vi "main.vi"() -> ()   [LabVIEW 2023]
uses:
  <vilib>/Analysis/1siggen.llb/Ramp Pattern by Samples.vi
  <vilib>/Analysis/NI_AALBase.lvlib
panel:
  in  "save":bool
  in  "Select temp":dbl=300.0 min=2.0 max=1800.0 format="%.2g"
  out "Signal (in uV/K)":dbl format="%.3g"
  out "S, -wire  /uV":dbl format="%.3g"
  out "S, +wire /uV":dbl format="%.3g"
  out "XY Graph":cluster{"temp /K":dbl[], "S_couple":dbl[]}[](graph)
  in  "Th  (Seebeck)":u16(ring)=5 caption="Thermocouple type" items=["B", "E", "J", "K", "R", "S", "T", "N"]
  in  "points":u16=100 min=1 max=2048
  in  "end temp /K":dbl=1273.0 min=2.0 max=1800.0 format="%#.2f"
  in  "start temp /K":dbl=273.0 min=2.0 max=1800.0 format="%#.2f"
  in  "exit":bool
  # "A simple program to calculate some Seebeck coefficients. Values taken from NIST monograph 175.\nN. Dragoe, Univ Paris-Saclay (first version LV8.6, may 2005. This version was compiled on 28/06/2025)."
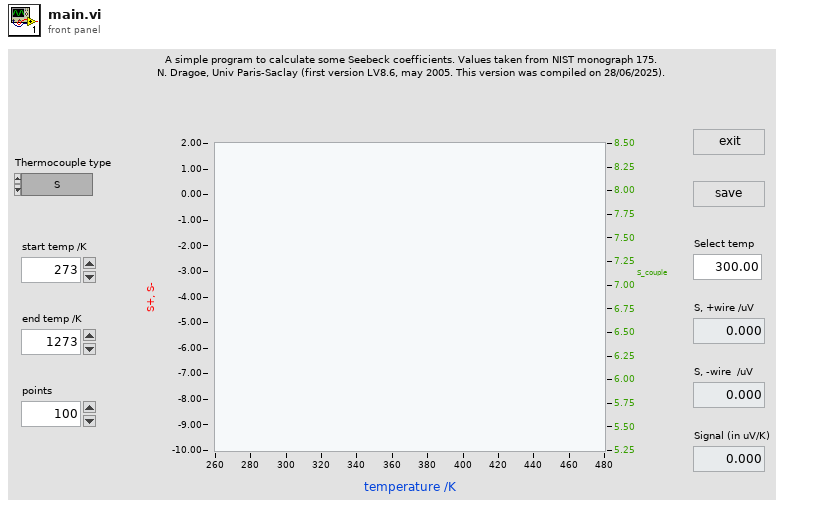
[diagram p1: front panel]
types:
  T1 = enum32{"Invalid", "Standard", "Closed", "Hidden", "Minimized", "Maximized"}
  T2 = enum32{"invalid app kind", "Development System", "Run Time System", "Student Edition", "Embedded LabVIEW", "Evaluation", "Custom"}
  T3 = cluster{"Core":cluster{"Current VI Reference":refnum<vi>, "Close Panel on Exit?":bool}, "Th  (Seebeck)":u16, "start temp /K":dbl, "end temp /K ":dbl, "points":u16, "S, -wire  /uV":dbl, "S, +wire /uV":dbl, "Signal (in uV/K)":dbl, "Select temp":dbl, "temp /K":dbl[], "S-":dbl[], "S+":dbl[], "S_couple":dbl[]}
  T4 = cluster{"Current VI Reference":refnum<vi>, "Close Panel on Exit?":bool}
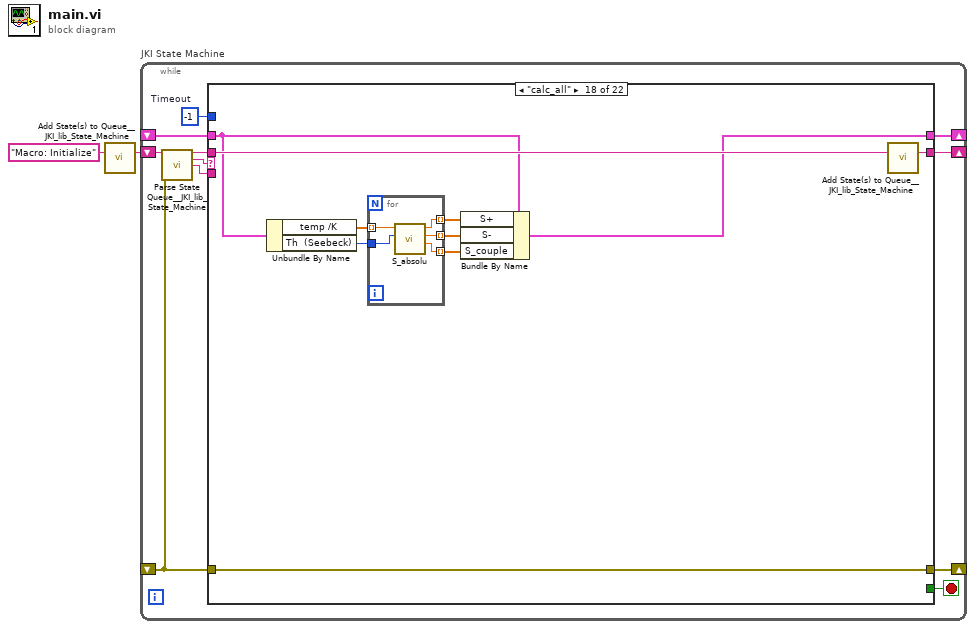
[diagram p0: block diagram]
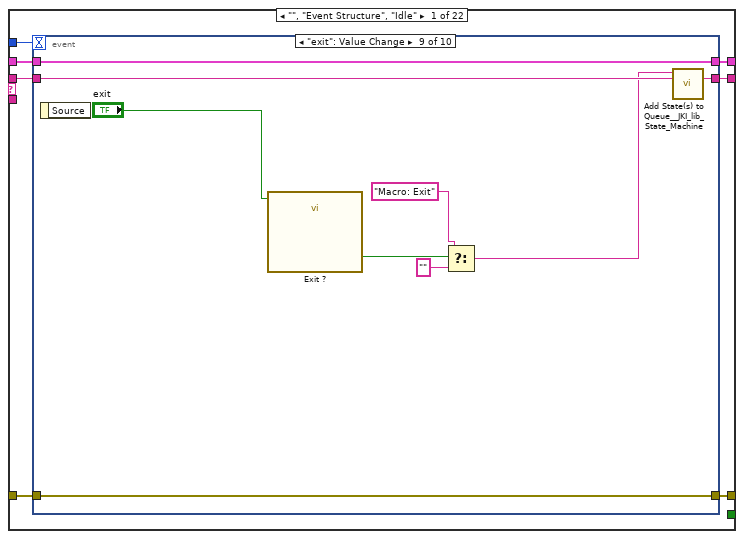
[diagram p2: hidden frame]
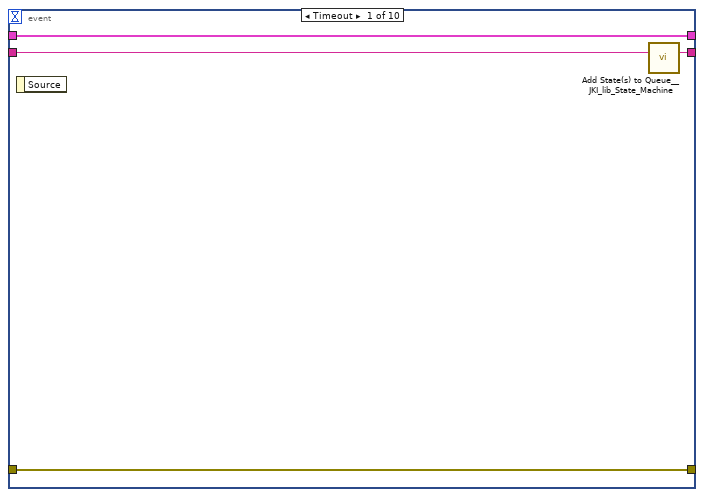
[diagram p3: hidden frame]
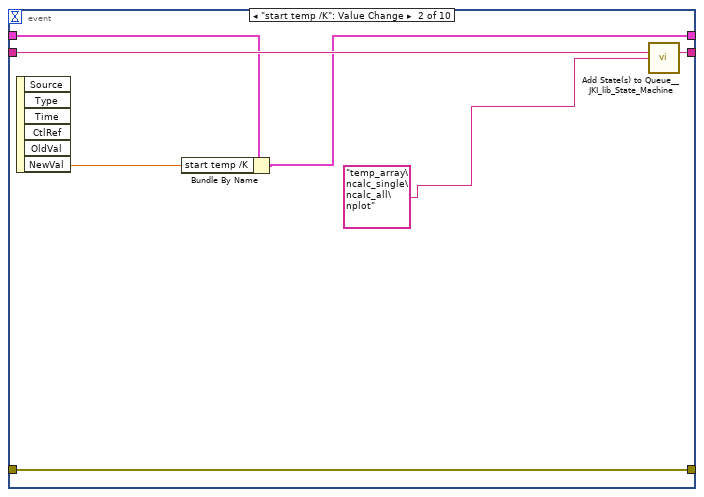
[diagram p4: hidden frame]
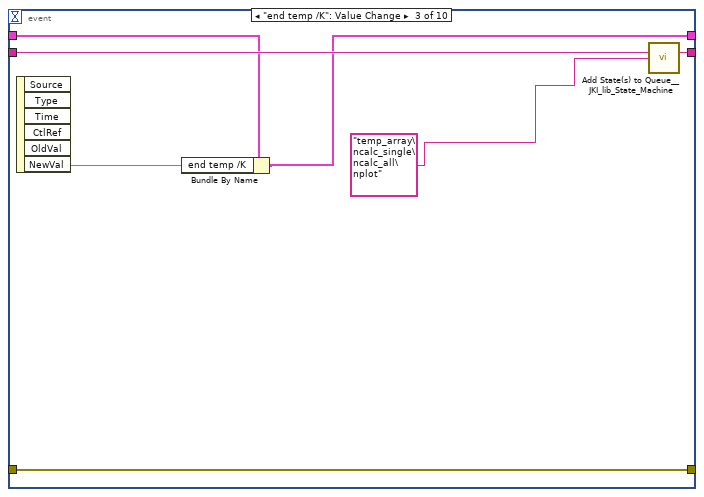
[diagram p5: hidden frame]
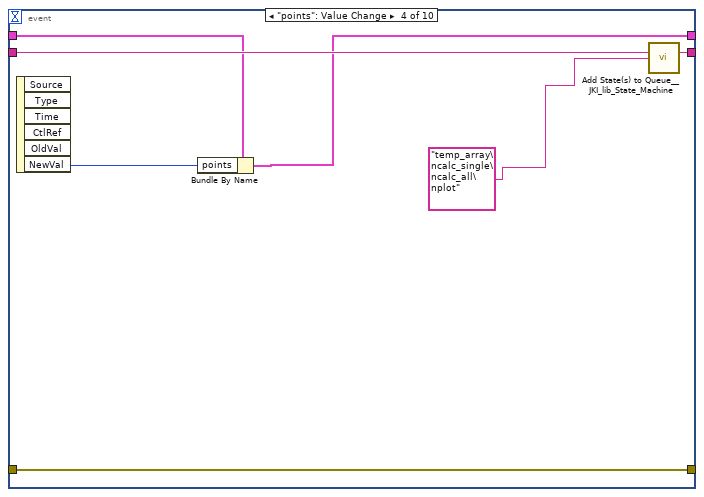
[diagram p6: hidden frame]
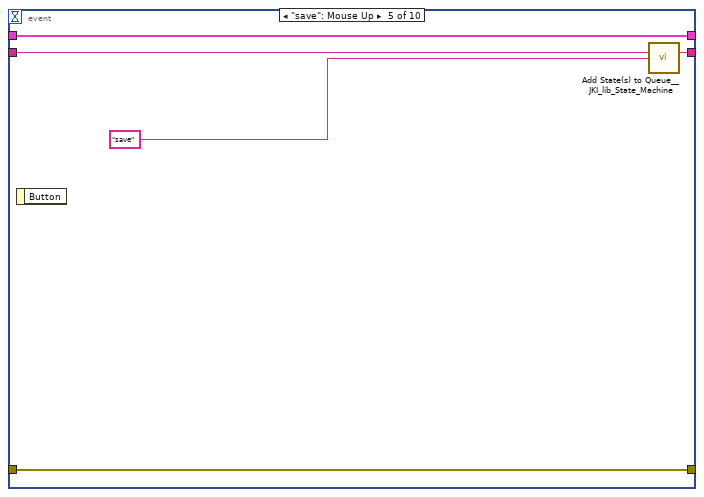
[diagram p7: hidden frame]
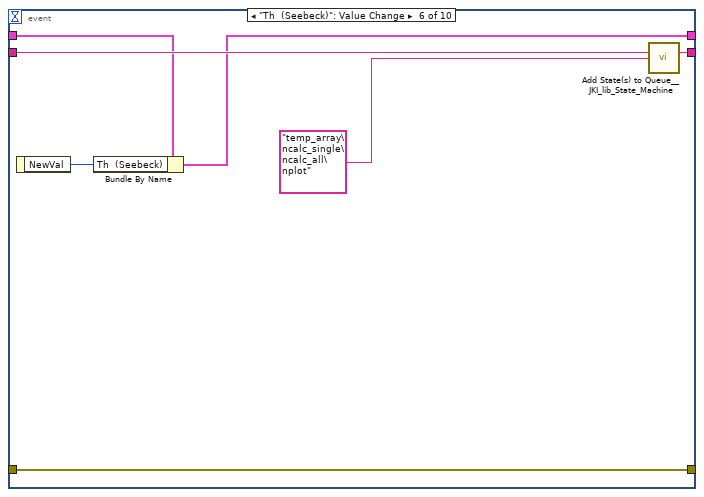
[diagram p8: hidden frame]
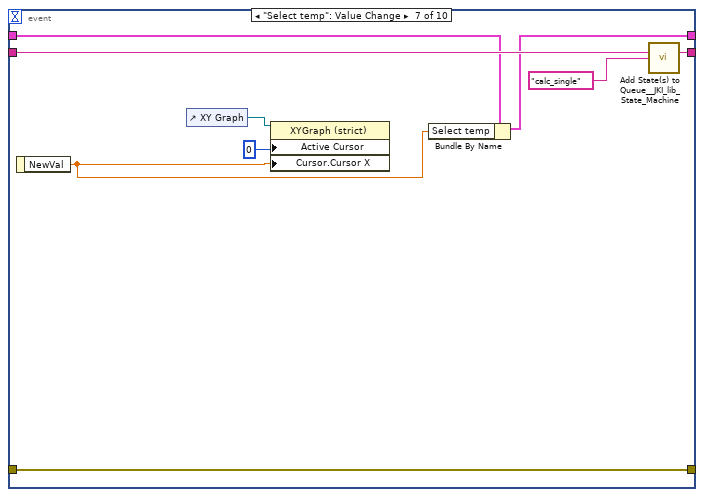
[diagram p9: hidden frame]
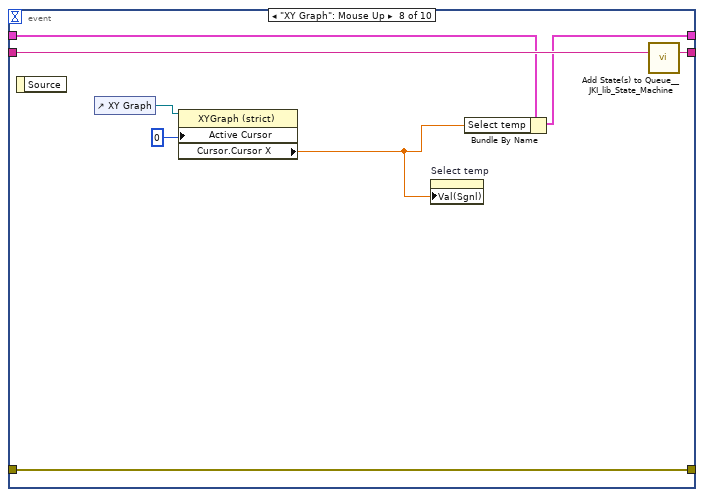
[diagram p10: hidden frame]
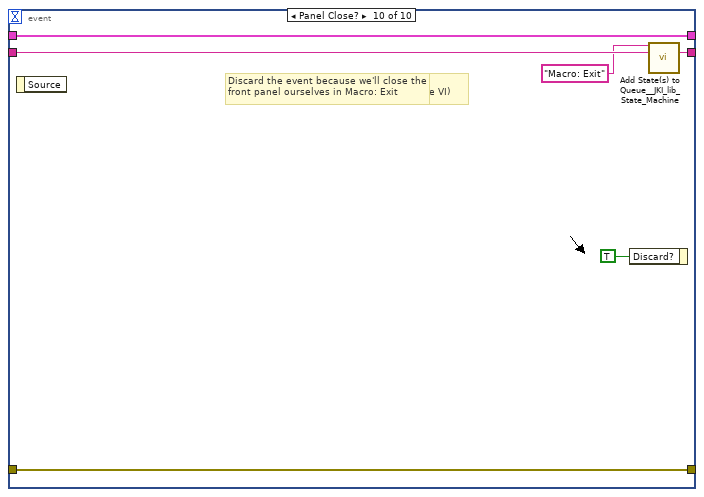
[diagram p11: hidden frame]
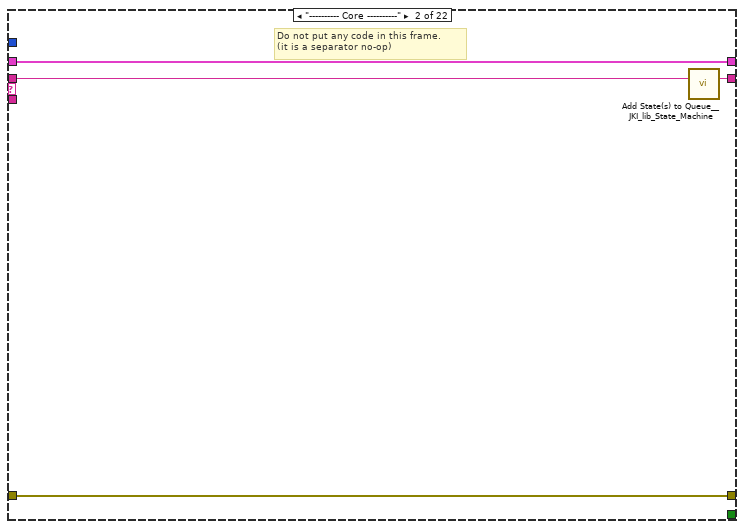
[diagram p12: hidden frame]
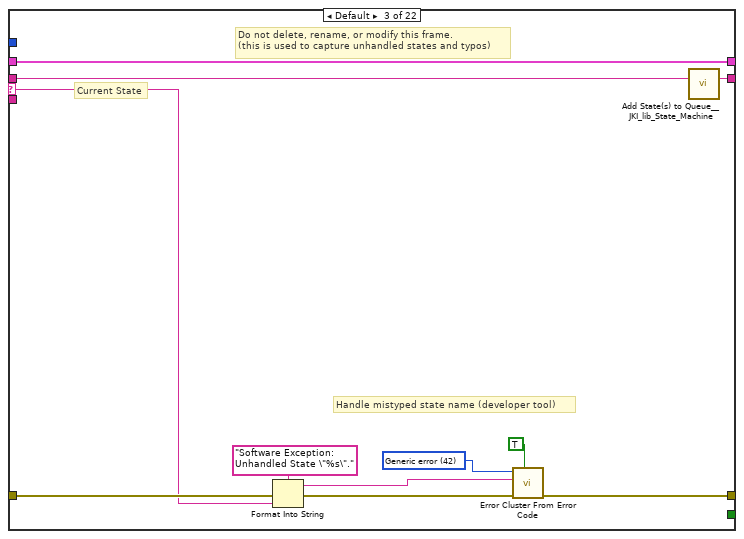
[diagram p13: hidden frame]
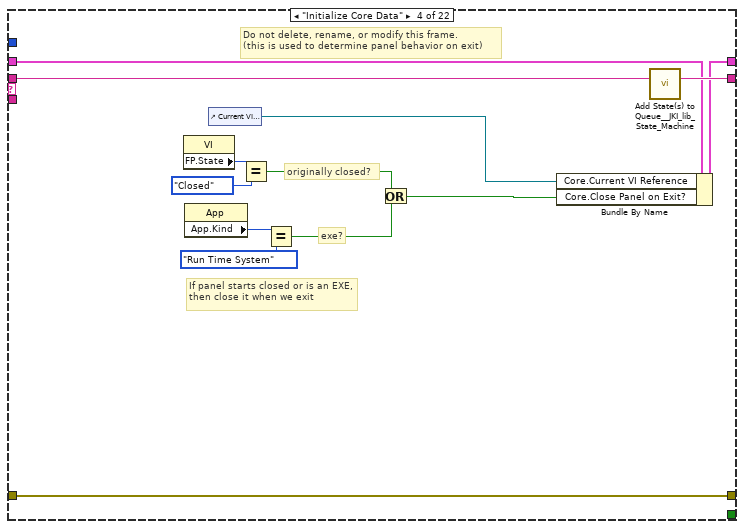
[diagram p14: hidden frame]
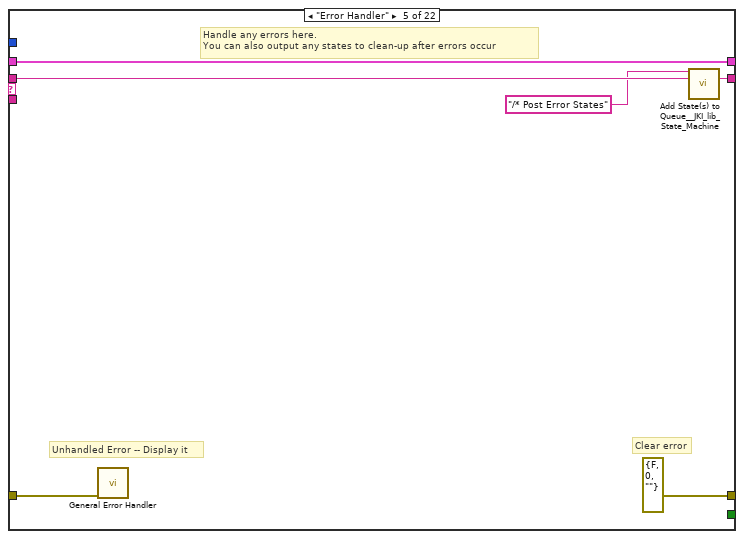
[diagram p15: hidden frame]
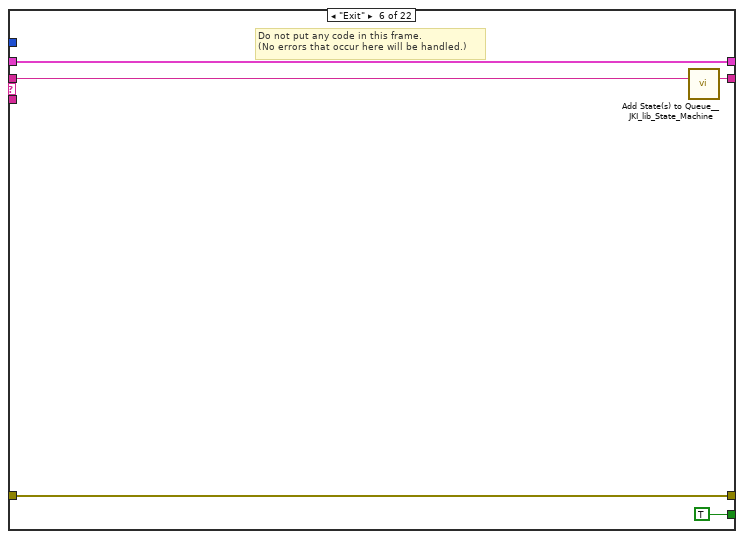
[diagram p16: hidden frame]
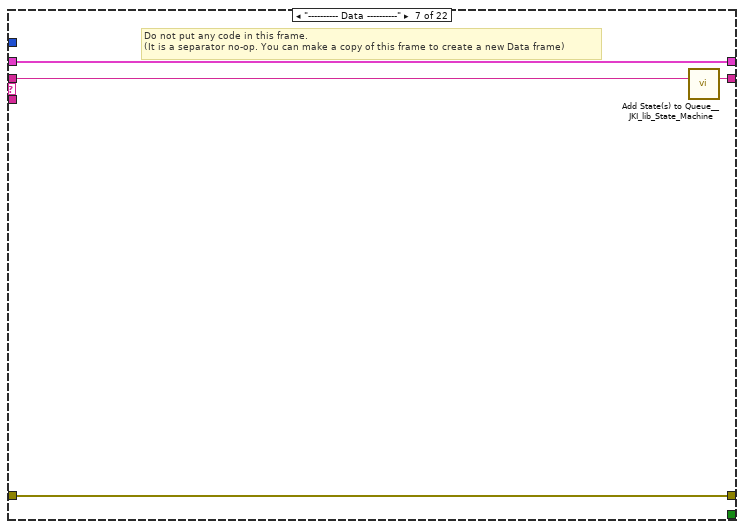
[diagram p17: hidden frame]
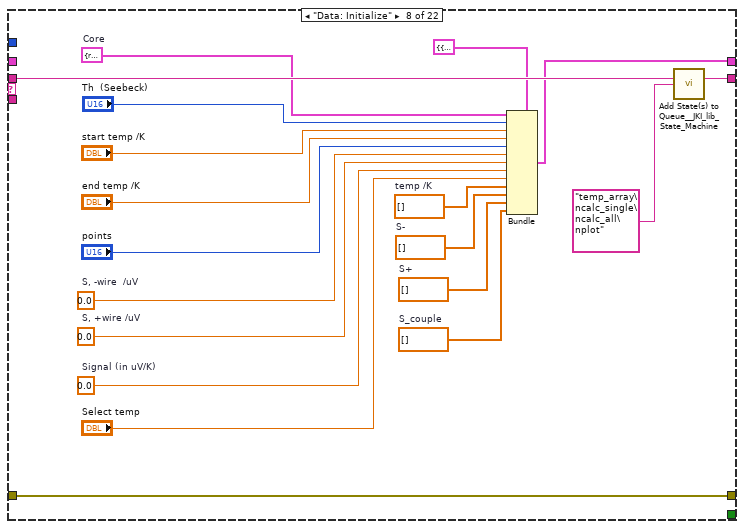
[diagram p18: hidden frame]
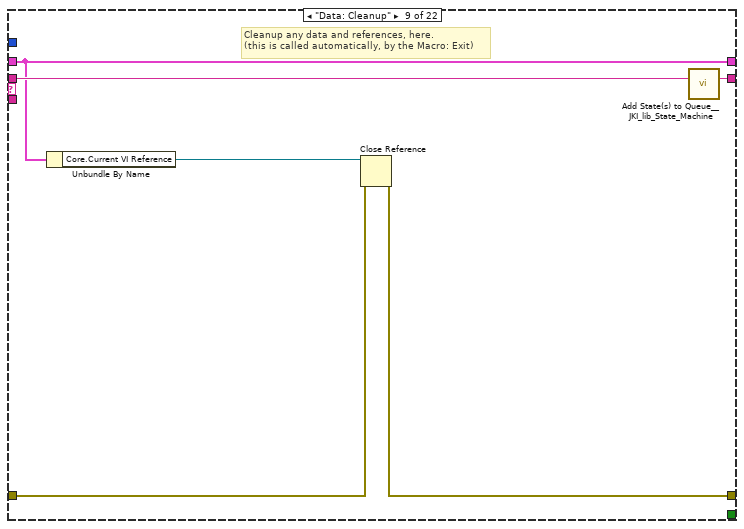
[diagram p19: hidden frame]
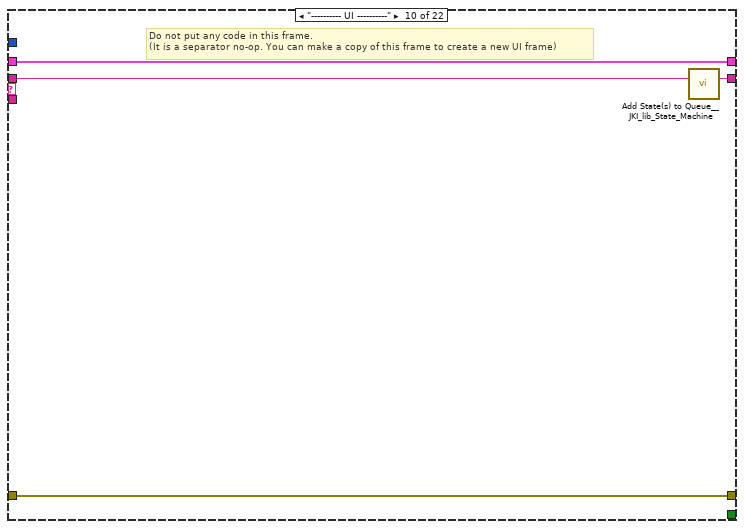
[diagram p20: hidden frame]
diagram:
  n1 = call <vilib>:"Add State(s) to Queue__JKI_lib_State_Machine.vi"("State(s) in (\"\")"="Macro: Initialize") -> ("States Out"=w2:string)  [unwired: 14 in]
  n2 = while "JKI State Machine" {
    shift-right: [w6] -> _
    shift-left: _ -> [w5]
    shift-right: [w9] -> _
    shift-left: _ -> [w3]
    shift-right: [w8] -> _
    shift-left: w2 -> [w10]
    stop <- w7 stop-if-true
    w4 = -1  # Timeout
    n3 = call <vilib>:"Parse State Queue__JKI_lib_State_Machine.vi"("State Queue"=w10, "Error In (no error)"=w3) -> ("Remaining States"=w12:string, "Current State"=w13:string, "Arguments"=w11:string)  [unwired: 11 in]
    n4 = case shown="\"calc_all\"" w13 {
      selector: w13 -> [_ _ w94 _ _ _ _ _ _ _ _ _ _ _ _ _ _ _ _ _ _ _]
      tunnel: w12 -> [w20 w93 w98 w117 w123 w128 w132 w151 w157 w161 w165 w171 w182 w251 w256 w266 w270 w280 w296 w305 w317 w335]
      tunnel: w11 -> [_ _ _ _ _ _ _ _ _ _ _ w166 w176 _ _ _ _ _ _ _ _ _]
      tunnel: w5 -> [w18 w90 w96 w110 w120 w126 w129 _ w152 w158 w163 w169 w178 w248 w253 w263 w267 w274 w286 w302 w314 w333]
      tunnel: [w17 w91 w100 w114 errorcluster {"status"=FALSE, "code"=0, "source"=""} ("error out") w125 w130 w149 w153 w159 w162 w167 w179 w249 w254 w264 w268 w278 w294 w303 w315 w332] -> w9
      tunnel: w3 -> [w16 w91 w99 w114 w119 w125 w130 w149 w154 w159 w162 w168 w180 w249 w254 w264 w268 w278 w294 w303 w315 w331]
      tunnel: [w19 w92 w97 w116 w122 w127 w131 w150 w156 w160 w164 w170 w181 w250 w255 w265 w269 w279 w295 w304 w316 w334] -> w8
      tunnel: [_ _ _ _ _ TRUE _ _ _ _ _ _ _ _ _ _ _ _ _ _ _ _] -> w7
      tunnel: [w15 w90 w96 w115 w120 w126 w129 w136 w152 w158 w163 w169 w178 w248 w253 w263 w267 w275 w287 w302 w314 w333] -> w6
      tunnel: w4 -> [w14 _ _ _ _ _ _ _ _ _ _ _ _ _ _ _ _ _ _ _ _ _]
      frame "", "Event Structure", "Idle" {
        n5 = event shown="[8] \"exit\": Value Change" {
          selector: _ -> [_ _ _ _ _ _ _ _ _ _]
          dyn-events: _ -> [_ _ _ _ _ _ _ _ _ _]
          timeout: w14 -> [_ _ _ _ _ _ _ _ _ _]
          tunnel: w20 -> [w24 w31 w38 w45 w50 w57 w66 w74 w83 w89]
          tunnel: [w23 w30 w37 w44 w49 w56 w65 w73 w82 w88] -> w19
          tunnel: w18 -> [w21 w26 w33 w40 w47 w52 w59 w68 w80 w86]
          tunnel: [w22 w29 w36 w43 w48 w55 w64 w72 w81 w87] -> w17
          tunnel: w16 -> [w22 w29 w36 w43 w48 w55 w64 w72 w81 w87]
          tunnel: [w21 w27 w34 w41 w47 w53 w60 w69 w80 w86] -> w15
          event Timeout {
            n6 = event-data() -> ()  [unwired: 1 in, 1 out]
            n7 = call <vilib>:"Add State(s) to Queue__JKI_lib_State_Machine.vi"("State(s) in (\"\")"=w24) -> ("States Out"=w23:string)  [unwired: 14 in]
          }
          event "start temp /K": Value Change {
            n8 = event-data() -> ("NewVal"=w28:dbl)  [unwired: 1 in, 5 out]
            n9 = Bundle By Name(cluster=w26, "start temp /K"=w28) -> (w27:T3)
            n10 = call <vilib>:"Add State(s) to Queue__JKI_lib_State_Machine.vi"("State(s) in (\"\")"=w31, "State(s) at Back (\"\")"="temp_array\ncalc_single\ncalc_all\nplot" ("State(s) at Back (\"\")")) -> ("States Out"=w30:string)  [unwired: 13 in]
          }
          event "end temp /K": Value Change {
            n11 = event-data() -> ("NewVal"=w35:dbl)  [unwired: 1 in, 5 out]
            n12 = Bundle By Name(cluster=w33, "end temp /K"=w35) -> (w34:T3)
            n13 = call <vilib>:"Add State(s) to Queue__JKI_lib_State_Machine.vi"("State(s) in (\"\")"=w38, "State(s) at Back (\"\")"="temp_array\ncalc_single\ncalc_all\nplot" ("State(s) at Back (\"\")")) -> ("States Out"=w37:string)  [unwired: 13 in]
          }
          event "points": Value Change {
            n14 = event-data() -> ("NewVal"=w42:u16)  [unwired: 1 in, 5 out]
            n15 = Bundle By Name(cluster=w40, "points"=w42) -> (w41:T3)
            n16 = call <vilib>:"Add State(s) to Queue__JKI_lib_State_Machine.vi"("State(s) in (\"\")"=w45, "State(s) at Back (\"\")"="temp_array\ncalc_single\ncalc_all\nplot" ("State(s) at Back (\"\")")) -> ("States Out"=w44:string)  [unwired: 13 in]
          }
          event "save": Mouse Up {
            n17 = event-data() -> ()  [unwired: 1 in, 1 out]
            n18 = call <vilib>:"Add State(s) to Queue__JKI_lib_State_Machine.vi"("State(s) in (\"\")"=w50, "State(s) at Back (\"\")"="save" ("State(s) at Back (\"\")")) -> ("States Out"=w49:string)  [unwired: 13 in]
          }
          event "Th  (Seebeck)": Value Change {
            n19 = event-data() -> ("NewVal"=w54:u16)  [unwired: 1 in]
            n20 = Bundle By Name(cluster=w52, "Th  (Seebeck)"=w54) -> (w53:T3)
            n21 = call <vilib>:"Add State(s) to Queue__JKI_lib_State_Machine.vi"("State(s) in (\"\")"=w57, "State(s) at Back (\"\")"="temp_array\ncalc_single\ncalc_all\nplot" ("State(s) at Back (\"\")")) -> ("States Out"=w56:string)  [unwired: 13 in]
          }
          event "Select temp": Value Change {
            n22 = event-data() -> ("NewVal"=w58:dbl)  [unwired: 1 in]
            n23 = control-ref of="XY Graph"() -> (w62:refnum<vi>)
            n24 = property on="Property Node" class="XYGraph (strict)"(reference=w62, "Active Cursor"=u32 0 ("Curseur actif"), "Cursor.Cursor X"=w58) -> ()  [unwired: 1 in, 2 out]
            n25 = Bundle By Name(cluster=w59, "Select temp"=w58) -> (w60:T3)
            n26 = call <vilib>:"Add State(s) to Queue__JKI_lib_State_Machine.vi"("State(s) in (\"\")"=w66, "State(s) at Back (\"\")"="calc_single" ("State(s) at Back (\"\")")) -> ("States Out"=w65:string)  [unwired: 13 in]
          }
          event "XY Graph": Mouse Up {
            n27 = event-data() -> ()  [unwired: 1 in, 1 out]
            n28 = control-ref of="XY Graph"() -> (w70:refnum<vi>)
            n29 = property on="Property Node" class="XYGraph (strict)"(reference=w70, "Active Cursor"=u32 0 ("Curseur actif")) -> ("Cursor.Cursor X"=w67:dbl)  [unwired: 1 in, 2 out]
            n30 = property on="Select temp" class="DigNum (strict)"("Val(Sgnl)"=w67) -> ()  [unwired: 2 in, 2 out]
            n31 = Bundle By Name(cluster=w68, "Select temp"=w67) -> (w69:T3)
            n32 = call <vilib>:"Add State(s) to Queue__JKI_lib_State_Machine.vi"("State(s) in (\"\")"=w74) -> ("States Out"=w73:string)  [unwired: 14 in]
          }
          event "exit": Value Change {
            n33 = event-data() -> ()  [unwired: 1 in, 1 out]
            n34 = call "Exit ?"("Enable"="exit") -> ("OK"=w78:bool)  [unwired: 17 in, 1 out]
            n35 = Select(t="Macro: Exit", s=w78, f="") -> (s? t:f=w76:string)
            n36 = call <vilib>:"Add State(s) to Queue__JKI_lib_State_Machine.vi"("State(s) in Front (\"\")"=w76, "State(s) in (\"\")"=w83) -> ("States Out"=w82:string)  [unwired: 13 in]
          }
          event Panel Close? {
            # "Discard the event because we'll close the front panel ourselves in Macro: Exit"
            # "Close Panel button (pressed) Event\n(this executes Macro: Exit to terminate the VI)"
            n37 = event-data() -> ()  [unwired: 1 in, 1 out]
            n38 = event-data("Discard?"=TRUE) -> ()  [unwired: 1 in, 1 out]
            n39 = call <vilib>:"Add State(s) to Queue__JKI_lib_State_Machine.vi"("State(s) in Front (\"\")"="Macro: Exit", "State(s) in (\"\")"=w89) -> ("States Out"=w88:string)  [unwired: 13 in]
          }
        }
      }
      frame "---------- Core ----------" {
        # "Do not put any code in this frame.\n(it is a separator no-op)"
        n40 = call <vilib>:"Add State(s) to Queue__JKI_lib_State_Machine.vi"("State(s) in (\"\")"=w93) -> ("States Out"=w92:string)  [unwired: 14 in]
      }
      frame Default {
        w103 = 42 items=["No error", "Argument error", "Memory is full", "Out of zone", "End of file", "File already open", "Generic file I/O error", "File not found", "File permission error", "Disk is full", "Duplicate path", "Too many files open", "System feature not enabled", "Resource file not found", "Cannot add resource", "Resource not found", "Image not found", "Image memory error", "Pen does not exist", "Config type invalid", "Config token not found", "Config parse error", "Config memory error", "Bad external code format", "Bad external code offset", "External code not present", "Null window", "Destroy window error", "Null menu", "Print aborted", "Bad print record", "Print driver error", "Windows error during printing", "Memory error during printing", "Print dialog error", "Generic print error", "Invalid device refnum", "Device not found", "Device parameter error", "Device unit error", "Cannot open device", "Device call aborted", "Generic error", "Cancelled by user", "Object ID too low", "Object ID too high", "Object not in heap", "Unknown heap", "Unknown object (invalid DefProc)", "Unknown object (DefProc not in table)", "Message out of range", "Invalid (null) method", "Unknown message", "Manager call not supported", "Bad address", "Network operation in progress", "Network operation timed out", "Connection is busy", "Network attribute not supported", "Network error", "Address in use", "System out of memory", "Connection aborted", "Connection refused", "Not connected", "Already connected", "Connection closed", "Initialization error (interapplication manager)", "Bad occurrence", "Wait on unbound occurrence handler", "Occurrence queue overflow", "Datalog type conflict", "Unused", "Unrecognized type (interapplication manager)", "Memory corrupt", "Failed to make temporary DLL", "Old CIN version", "Drag socket not found", "Failed to load drop-object", "Failed to register OLE object", "Failed to release OLE object", "Format specifier type mismatch", "Unknown format specifier", "Too few format specifiers", "Too many format specifiers", "Scan failed", "Newer CIN version", "Error converting to variant", "Runtime menu error", "Password tampered", "Variant attribute not found", "Incompatible variant data type", "Event data is not available", "Event Store is not present", "Occurrence is not found", "Event Queue is not created", "Event info is not available", "Refnum passed is NULL", "Error retrieving Class GUID", "Error retrieving CoClass GUID", "Error retrieving TypeLib GUID.", "Bad built application magic bytes.", "Specific driver is different from the specific driver associated with the Logical Name.", "There is no session opened to the class driver.", "Max Error", "MAX - Error with config objects", "MAX - Error loading configuration", "MAX - Group not supported"]
        # "Current State"
        # "Do not delete, rename, or modify this frame.\n(this is used to capture unhandled states and typos)"
        # "Handle mistyped state name (developer tool)"
        n41 = Format Into String(format string="Software Exception: Unhandled State \"%s\"." ("message"), error in=w99, w94) -> (resulting string=w102:string, error out=w101:errorcluster)  [unwired: 1 in]
        n42 = call <vilib>:"Error Cluster From Error Code.vi"("show call chain? (False)"=TRUE, "error in (no error)"=w101, "error message (\"\")"=w102, "error code (0)"=w103) -> ("error out"=w100:errorcluster)  [unwired: 5 in]
        n43 = call <vilib>:"Add State(s) to Queue__JKI_lib_State_Machine.vi"("State(s) in (\"\")"=w98) -> ("States Out"=w97:string)  [unwired: 14 in]
      }
      frame "Initialize Core Data" {
        # "Do not delete, rename, or modify this frame.\n(this is used to determine panel behavior on exit)"
        # "originally closed?"
        # "exe?"
        # "If panel starts closed or is an EXE, then close it when we exit"
        n44 = property class="VI"() -> ("FP.State"=w107:T1)  [unwired: 2 in, 2 out]
        n45 = property class="App"() -> ("App.Kind"=w113:T2)  [unwired: 2 in, 2 out]
        n46 = control-ref of="Current VI Reference"() -> (w108:refnum<vi>)
        n47 = Equal?(x=w107, y=T1."Closed" ("Front Panel Window:State")) -> (x = y?=w105:bool)
        n48 = Equal?(x=w113, y=T2."Run Time System" ("Application:Kind")) -> (x = y?=w111:bool)
        n49 = Or(x=w105, y=w111) -> (x .or. y?=w109:bool)
        n50 = Bundle By Name(cluster=w110, "Core.Current VI Reference"=w108, "Core.Close Panel on Exit?"=w109) -> (w115:T3)
        n51 = call <vilib>:"Add State(s) to Queue__JKI_lib_State_Machine.vi"("State(s) in (\"\")"=w117) -> ("States Out"=w116:string)  [unwired: 14 in]
      }
      frame "Error Handler" {
        # "Unhandled Error -- Display it"
        # "Handle any errors here.\nYou can also output any states to clean-up after errors occur"
        # "Clear error"
        n52 = call <vilib>:"General Error Handler.vi"("error in (no error)"=w119) -> ()  [unwired: 10 in, 5 out]
        n53 = call <vilib>:"Add State(s) to Queue__JKI_lib_State_Machine.vi"("State(s) in Front (\"\")"="/* Post Error States", "State(s) in (\"\")"=w123) -> ("States Out"=w122:string)  [unwired: 13 in]
      }
      frame "Exit" {
        # "Do not put any code in this frame.\n(No errors that occur here will be handled.)"
        n54 = call <vilib>:"Add State(s) to Queue__JKI_lib_State_Machine.vi"("State(s) in (\"\")"=w128) -> ("States Out"=w127:string)  [unwired: 14 in]
      }
      frame "---------- Data ----------" {
        # "Do not put any code in this frame.\n(It is a separator no-op. You can make a copy of this frame to create a new Data frame)"
        n55 = call <vilib>:"Add State(s) to Queue__JKI_lib_State_Machine.vi"("State(s) in (\"\")"=w132) -> ("States Out"=w131:string)  [unwired: 14 in]
      }
      frame "Data: Initialize" {
        w137 = dbl[] []  # S_couple
        w138 = dbl[] []  # S+
        w139 = dbl[] []  # S-
        w140 = dbl[] []  # temp /K
        w143 = 0.0  # Signal (in uV/K)
        w144 = 0.0  # S, +wire /uV
        w145 = 0.0  # S, -wire  /uV
        w148 = T4 {"Current VI Reference"=refnum, "Close Panel on Exit?"=FALSE}  # Core
        n56 = Bundle(cluster=T3 {"Core"={"Current VI Reference"=refnum, "Close Panel on Exit?"=FALSE}, "Th  (Seebeck)"=0, "start temp /K"=0.0, "end temp /K "=0.0, "points"=0, "S, -wire  /uV"=0.0, "S, +wire /uV"=0.0, "Signal (in uV/K)"=0.0, "Select temp"=0.0, "temp /K"=[], "S-"=[], "S+"=[], "S_couple"=[]}, "Core"=w148, "Th  (Seebeck)"="Th  (Seebeck)", "start temp /K"="start temp /K", "end temp /K"="end temp /K", "points"="points", "S, -wire  /uV"=w145, "S, +wire /uV"=w144, "Signal (in uV/K)"=w143, "Select temp"="Select temp", "temp /K"=w140, "S-"=w139, "S+"=w138, "S_couple"=w137) -> (w136:T3)
        n57 = call <vilib>:"Add State(s) to Queue__JKI_lib_State_Machine.vi"("State(s) in (\"\")"=w151, "State(s) at Back (\"\")"="temp_array\ncalc_single\ncalc_all\nplot" ("State(s) at Back (\"\")")) -> ("States Out"=w150:string)  [unwired: 13 in]
      }
      frame "Data: Cleanup" {
        # "Cleanup any data and references, here.\n(this is called automatically, by the Macro: Exit)"
        n58 = Unbundle By Name(w152) -> ("Core.Current VI Reference"=w155:refnum<vi>)
        n59 = Close Reference(reference=w155, error in (no error)=w154) -> (error out=w153:errorcluster)
        n60 = call <vilib>:"Add State(s) to Queue__JKI_lib_State_Machine.vi"("State(s) in (\"\")"=w157) -> ("States Out"=w156:string)  [unwired: 14 in]
      }
      frame "---------- UI ----------" {
        # "Do not put any code in this frame.\n(It is a separator no-op. You can make a copy of this frame to create a new UI frame)"
        n61 = call <vilib>:"Add State(s) to Queue__JKI_lib_State_Machine.vi"("State(s) in (\"\")"=w161) -> ("States Out"=w160:string)  [unwired: 14 in]
      }
      frame "UI: Initialize" {
        # "Initialize the User Interface, here.\n(this is called automatically, by the Macro: Init)"
        n62 = call <vilib>:"Add State(s) to Queue__JKI_lib_State_Machine.vi"("State(s) in (\"\")"=w165) -> ("States Out"=w164:string)  [unwired: 14 in]
      }
      frame "UI: Cursor Set" {
        # "Argument"
        # "Set and Unset Cursor Busy.\n(Usage: \"UI: Cursor Set >> Busy|Idle\")"
        n63 = case shown="\"Idle\", Default" w166 {
          tunnel: w168 -> [w173 w175]
          tunnel: [w172 w174] -> w167
          frame "Idle", Default {
            n64 = call <vilib>:"Unset Busy.vi"("error in (no error)"=w173) -> ("error out"=w172:errorcluster)  [unwired: 10 in]
          }
          frame "Busy" {
            n65 = call <vilib>:"Set Busy.vi"("error in (no error)"=w175) -> ("error out"=w174:errorcluster)  [unwired: 9 in, 1 out]
          }
        }
        n66 = call <vilib>:"Add State(s) to Queue__JKI_lib_State_Machine.vi"("State(s) in (\"\")"=w171) -> ("States Out"=w170:string)  [unwired: 14 in]
      }
      frame "UI: Front Panel State" {
        # "Argument"
        # "Set Front Panel Open or Closed\n(Usage: \"UI: Front Panel State >> Open|Close\")"
        n67 = Unbundle By Name(w178) -> ("Core.Current VI Reference"=w177:refnum<vi>)
        n68 = case shown="\"Minimize\", \"Minimized\"" w176 {
          tunnel: w180 -> [w188 w203 w214 w227 w240]
          tunnel: [w190 w204 w216 w229 w242] -> w179
          tunnel: w177 -> [w189 w201 w215 w228 w241]
          frame "Open", "Standard", Default {
            w183 = T1."Standard" ("State")
            n69 = property class="VI"(reference=w189, error in=w188) -> (reference out=w186:refnum<vi>, error out=w187:errorcluster, "FP.State"=w185:T1)
            n70 = Not Equal?(x=w185, y=w183) -> (x != y?=w184:bool)
            n71 = case shown="True" w184 {
              tunnel: [w194 w196] -> w190
              tunnel: w187 -> [w193 w196]
              tunnel: w186 -> [w192 _]
              tunnel: w183 -> [w191 _]
              frame True {
                n72 = invoke class="VI" method="FP.Open"(reference=w192, error in=w193, "Activate"=TRUE, "State"=w191) -> (error out=w194:errorcluster)  [unwired: 1 in, 4 out]
              }
              frame False {
              }
            }
          }
          frame "Close", "Closed" {
            n73 = property class="VI"(reference=w201, error in=w203) -> (reference out=w200:refnum<vi>, error out=w202:errorcluster, "FP.State"=w198:T1)
            n74 = Not Equal?(x=w198, y=T1."Closed" ("Front Panel Window:State")) -> (x != y?=w197:bool)
            n75 = case shown="True" w197 {
              tunnel: [w205 w208] -> w204
              tunnel: w202 -> [w205 w207]
              tunnel: w200 -> [_ w206]
              frame False {
              }
              frame True {
                n76 = invoke class="VI" method="FP.Close"(reference=w206, error in=w207) -> (error out=w208:errorcluster)  [unwired: 1 in, 2 out]
              }
            }
          }
          frame "Hidden", "Hide" {
            w209 = T1."Hidden" ("State")
            n77 = property class="VI"(reference=w215, error in=w214) -> (reference out=w212:refnum<vi>, error out=w213:errorcluster, "FP.State"=w211:T1)
            n78 = Not Equal?(x=w211, y=w209) -> (x != y?=w210:bool)
            n79 = case shown="True" w210 {
              tunnel: [w220 w221] -> w216
              tunnel: w213 -> [w219 w221]
              tunnel: w212 -> [w218 _]
              tunnel: w209 -> [w217 _]
              frame True {
                n80 = invoke class="VI" method="FP.Open"(reference=w218, error in=w219, "State"=w217) -> (error out=w220:errorcluster)  [unwired: 2 in, 4 out]
              }
              frame False {
              }
            }
          }
          frame "Minimize", "Minimized" {
            w222 = T1."Minimized" ("State")
            n81 = property class="VI"(reference=w228, error in=w227) -> (reference out=w225:refnum<vi>, error out=w226:errorcluster, "FP.State"=w224:T1)
            n82 = Not Equal?(x=w224, y=w222) -> (x != y?=w223:bool)
            n83 = case shown="True" w223 {
              tunnel: [w233 w234] -> w229
              tunnel: w226 -> [w232 w234]
              tunnel: w225 -> [w231 _]
              tunnel: w222 -> [w230 _]
              frame True {
                n84 = invoke class="VI" method="FP.Open"(reference=w231, error in=w232, "State"=w230) -> (error out=w233:errorcluster)  [unwired: 2 in, 4 out]
              }
              frame False {
              }
            }
          }
          frame "Maximize", "Maximized" {
            w235 = T1."Maximized" ("State")
            n85 = property class="VI"(reference=w241, error in=w240) -> (reference out=w238:refnum<vi>, error out=w239:errorcluster, "FP.State"=w237:T1)
            n86 = Not Equal?(x=w237, y=w235) -> (x != y?=w236:bool)
            n87 = case shown="True" w236 {
              tunnel: [w246 w247] -> w242
              tunnel: w239 -> [w245 w247]
              tunnel: w238 -> [w244 _]
              tunnel: w235 -> [w243 _]
              frame True {
                n88 = invoke class="VI" method="FP.Open"(reference=w244, error in=w245, "State"=w243) -> (error out=w246:errorcluster)  [unwired: 2 in, 4 out]
              }
              frame False {
              }
            }
          }
        }
        n89 = call <vilib>:"Add State(s) to Queue__JKI_lib_State_Machine.vi"("State(s) in (\"\")"=w182) -> ("States Out"=w181:string)  [unwired: 14 in]
      }
      frame "---------- Macro ----------" {
        # "Do not put any code in this frame.\n(It is a separator no-op. You can make a copy of this frame to create a new Macro frame)"
        n90 = call <vilib>:"Add State(s) to Queue__JKI_lib_State_Machine.vi"("State(s) in (\"\")"=w251) -> ("States Out"=w250:string)  [unwired: 14 in]
      }
      frame "Macro: Initialize" {
        w252 = "Data: Initialize\nInitialize Core Data\nUI: Initialize\nUI: Front Panel State >> Open"  # Data: Initialize Initialize Core Data UI: Initialize UI: Front Panel State >> Open
        n91 = call <vilib>:"Add State(s) to Queue__JKI_lib_State_Machine.vi"("State(s) in Front (\"\")"=w252, "State(s) in (\"\")"=w256) -> ("States Out"=w255:string)  [unwired: 13 in]
      }
      frame "Macro: Exit" {
        # "Exit Macro\n(This is called once, when the VI exits)"
        n92 = Unbundle By Name(w263) -> ("Core.Close Panel on Exit?"=w262:bool)
        n93 = Select(t="UI: Front Panel State >> Close", s=w262, f="") -> (s? t:f=w259:string)
        n94 = call <vilib>:"Add State(s) to Queue__JKI_lib_State_Machine.vi"("State(s) in (\"\")"=w259, "State(s) at Back (\"\")"="Data: Cleanup\nExit") -> ("States Out"=w257:string)  [unwired: 13 in]
        n95 = call <vilib>:"Add State(s) to Queue__JKI_lib_State_Machine.vi"("State(s) in Front (\"\")"=w257, "State(s) in (\"\")"=w266) -> ("States Out"=w265:string)  [unwired: 13 in]
      }
      frame "---------- Calc ----------" {
        n96 = call <vilib>:"Add State(s) to Queue__JKI_lib_State_Machine.vi"("State(s) in (\"\")"=w270) -> ("States Out"=w269:string)  [unwired: 14 in]
      }
      frame "calc_all" {
        n97 = Unbundle By Name(w274) -> ("temp /K"=w277:dbl[], "Th  (Seebeck)"=w276:u16)
        n98 = for {
          tunnel: w277 -> [w285] mode=indexing
          tunnel: w276 -> [w284]
          tunnel: [w283] -> w273 mode=indexing
          tunnel: [w282] -> w272 mode=indexing
          tunnel: [w281] -> w271 mode=indexing
          n99 = call "S_absolu.vi"("Th  (Seebeck)"=w284, "T, in  Kelvin"=w285) -> ("TC signal /microVperK"=w281:dbl, "S of - wire /microV/K"=w282:dbl, "S of + wire /microV/K"=w283:dbl)  [unwired: 7 in]
        }
        n100 = Bundle By Name(cluster=w274, "S+"=w273, "S-"=w272, "S_couple"=w271) -> (w275:T3)
        n101 = call <vilib>:"Add State(s) to Queue__JKI_lib_State_Machine.vi"("State(s) in (\"\")"=w280) -> ("States Out"=w279:string)  [unwired: 14 in]
      }
      frame "temp_array" {
        w289 = u16 0 items=["Linear", "Logarithmic"] ("type")
        n102 = Unbundle By Name(w286) -> ("points"=w293:u16, "end temp /K"=w292:dbl, "start temp /K"=w291:dbl)  [unwired: 1 out]
        n103 = call-poly <vilib>:"Ramp Pattern.vi"("type"=w289, "exclude end?"=FALSE, "start"=w291, "end"=w292, "samples"=w293) -> ("Ramp Pattern"=w288:dbl[])  [unwired: 5 in, 1 out]
        n104 = Bundle By Name(cluster=w286, "temp /K"=w288) -> (w287:T3)
        n105 = call <vilib>:"Add State(s) to Queue__JKI_lib_State_Machine.vi"("State(s) in (\"\")"=w296) -> ("States Out"=w295:string)  [unwired: 14 in]
      }
      frame "calc_single" {
        n106 = Unbundle By Name(w302) -> ("Select temp"=w301:dbl, "Th  (Seebeck)"=w300:u16)
        n107 = call "S_absolu.vi"("Th  (Seebeck)"=w300, "T, in  Kelvin"=w301) -> ("TC signal /microVperK"=→"Signal (in uV/K)":dbl, "S of - wire /microV/K"=→"S, -wire  /uV":dbl, "S of + wire /microV/K"=→"S, +wire /uV":dbl)  [unwired: 7 in]
        n108 = call <vilib>:"Add State(s) to Queue__JKI_lib_State_Machine.vi"("State(s) in (\"\")"=w305) -> ("States Out"=w304:string)  [unwired: 14 in]
      }
      frame "plot" {
        n109 = Unbundle By Name(w314) -> ("temp /K"=w311:dbl[], "S-"=w313:dbl[], "S+"=w312:dbl[], "S_couple"=w310:dbl[])
        n110 = Bundle("temp /K"=w311, "S-"=w313) -> (w309:cluster{"temp /K":dbl[], "S-":dbl[]})  [unwired: 1 in]
        n111 = Bundle("temp /K"=w311, "S+"=w312) -> (w308:cluster{"temp /K":dbl[], "S+":dbl[]})  [unwired: 1 in]
        n112 = Bundle("temp /K"=w311, "S_couple"=w310) -> (w307:cluster{"temp /K":dbl[], "S_couple":dbl[]})  [unwired: 1 in]
        n113 = Build Array(w309, w308, w307) -> (→"XY Graph":cluster{"temp /K":dbl[], "S_couple":dbl[]}[])
        n114 = call <vilib>:"Add State(s) to Queue__JKI_lib_State_Machine.vi"("State(s) in (\"\")"=w317) -> ("States Out"=w316:string)  [unwired: 14 in]
      }
      frame "save" {
        n115 = Unbundle By Name(w333) -> ("Th  (Seebeck)"=w320:u16, "temp /K"=w330:dbl[], "S-"=w329:dbl[], "S+"=w328:dbl[], "S_couple"=w327:dbl[])
        n116 = property on="Th  (Seebeck)" class="Ring (strict)"() -> ("Strings []"=w321:string[])  [unwired: 2 in, 2 out]
        n117 = for {
          tunnel: w330 -> [w345] mode=indexing
          tunnel: w329 -> [w344] mode=indexing
          tunnel: w328 -> [w343] mode=indexing
          tunnel: w327 -> [w342] mode=indexing
          tunnel: [w336] -> w326 mode=indexing
          w337 = "\t"
          n118 = Number To Exponential String(number=w345) -> (E-format string=w341:string)  [unwired: 3 in]
          n119 = Number To Exponential String(number=w344) -> (E-format string=w340:string)  [unwired: 3 in]
          n120 = Number To Exponential String(number=w343) -> (E-format string=w339:string)  [unwired: 3 in]
          n121 = Number To Exponential String(number=w342) -> (E-format string=w338:string)  [unwired: 3 in]
          n122 = Concatenate Strings(w341, w337, w340, w337, w339, w337, w338) -> (w336:string)
        }
        n123 = Index Array(array=w321, index=w320) -> (element=w318:string)
        n124 = Concatenate Strings("Thermocouple type: " ("E-format string"), w318, "\r\n", "Temp /K, S-/uV, S+/uV, S couple/uV" ("E-format string")) -> (w322:string)
        n125 = Build Array (concatenate)(w322, w326) -> (w325:string[])
        n126 = Write to Text File(text=w325, error in=w331) -> (error out=w332:errorcluster)  [unwired: 2 in, 2 out]
        n127 = call <vilib>:"Add State(s) to Queue__JKI_lib_State_Machine.vi"("State(s) in (\"\")"=w335) -> ("States Out"=w334:string)  [unwired: 14 in]
      }
    }
  }
